vi "reportAllFAADCScanRate.vi"(8 "error in (no error)":errorcluster, 10 "ModbusBuffer in":refnum<class "ModbusBuffer.lvclass">, 11 "ILCCommunications in":refnum<class "ILCCommunications.lvclass">) -> (0 "error out":errorcluster, 2 "ModbusBuffer out":refnum<class "ModbusBuffer.lvclass">, 3 "ILCCommunications out":refnum<class "ILCCommunications.lvclass">)   [LabVIEW 2016, in "ILCCommunications.lvclass"]
uses:
  ILCCommunications.lvclass
  Common_RT_Modbus/ModbusBuffer/ModbusBuffer.lvclass
  ILCCommunications.lvclass/ILCCommunications.ctl
  Common_RT_ILC/ILC/ILC.lvclass/ILC.ctl
  Common_RT_Modbus/ModbusBuffer/ModbusBuffer.lvclass/ModbusBuffer.ctl
  reportADCScanRate.vi
  Common_RT_ILC/ILC/addADCScanRateFrame.vi
  Common_RT_ILC/ILC/getILCData.vi
  Common_RT_ILC/ILC/setILCData.vi
  Common_RT_Modbus/ModbusBuffer/writeHeader.vi
  Common_RT_Modbus/ModbusBuffer/writeU8.vi
  Common_RT_Modbus/ModbusBuffer/writeCRC.vi
  Common_RT_Modbus/ModbusBuffer/writeEndOfFrame.vi
  Common_RT_Modbus/ModbusBuffer/writeWaitForRx.vi
  Common_RT_Modbus/ModbusBuffer/writeByteInstruction.vi
  Common_RT_Modbus/ModbusBuffer/calculateCRC.vi
  Common_RT_FAILC/FAILC/FAILC.lvclass
  D:/Code/ts_M1M3Support/Common_RT_ILC/ILC/ILC.lvclass
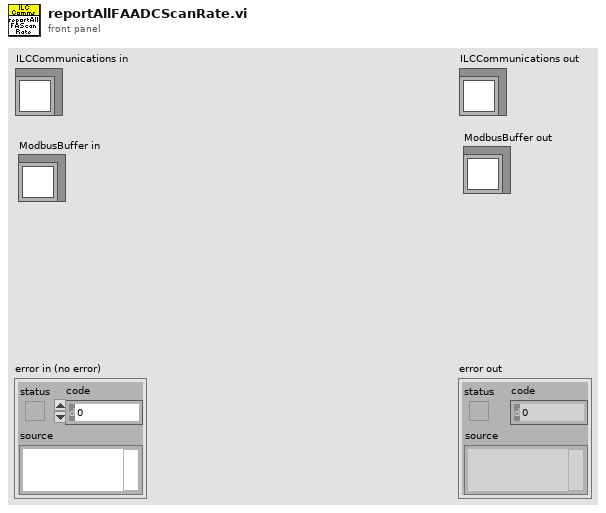
[diagram p1: front panel]
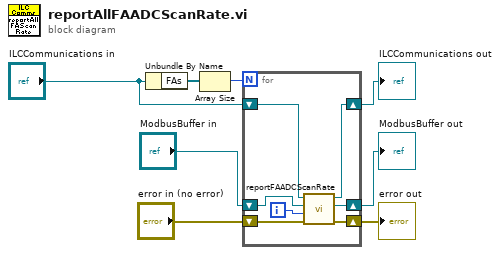
[diagram p0: block diagram]
diagram:
  n1 = Unbundle By Name("ILCCommunications in") -> ("FAs"=w8:refnum<class "FAILC.lvclass">[])
  n2 = Array Size(array=w8) -> (size(s)=w6:i32)
  n3 = for {
    N: w6 -> [_]
    shift-right: [w13] -> w5
    shift-left: "ILCCommunications in" -> [w15]
    shift-right: [w14] -> w3
    shift-left: "error in (no error)" -> [w12]
    shift-right: [w9] -> w1
    shift-left: "ModbusBuffer in" -> [w10]
    i -> [w11]
    n4 = call "reportFAADCScanRate.vi"("error in (no error)"=w12, "FAIndex"=w11, "ModbusBuffer in"=w10, "ILCCommunications in"=w15) -> ("error out"=w14:errorcluster, "ModbusBuffer out"=w9:refnum<class "ModbusBuffer.lvclass">, "ILCCommunications out"=w13:refnum<class "ILCCommunications.lvclass">)  [unwired: 5 in]
  }
  "error out" <- w3
  "ILCCommunications out" <- w5
  "ModbusBuffer out" <- w1
